vi "UpdateSpeeds.vi"(4 "SpeedMutiplier":dbl=2.0, 6 "Ramp (V/s)":dbl=2.0, 7 "robotPositionIn":T1, 8 "Enabled":bool=TRUE, 9 "Rotation (V)":dbl, 10 "Left/Right (V)":dbl, 11 "Forwards/Back (V)":dbl) -> (0 "M4 (V)":dbl, 1 "M3 (V)":dbl, 2 "M2 (V)":dbl, 3 "M1 (V)":dbl, 5 "robotPositionOut":T1)   [LabVIEW 2015]
panel:
  out "Distance Travelled (mm/0.01s)":dbl
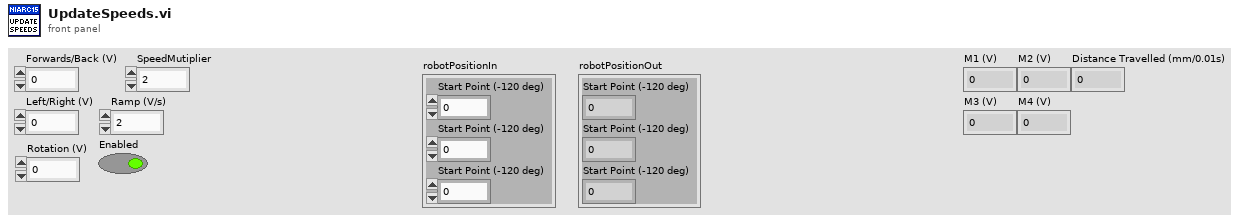
[diagram p1: front panel]
types:
  T1 = cluster{"Start Point (-120 deg)":dbl, "Start Point (-120 deg)":dbl, "Start Point (-120 deg)":dbl}
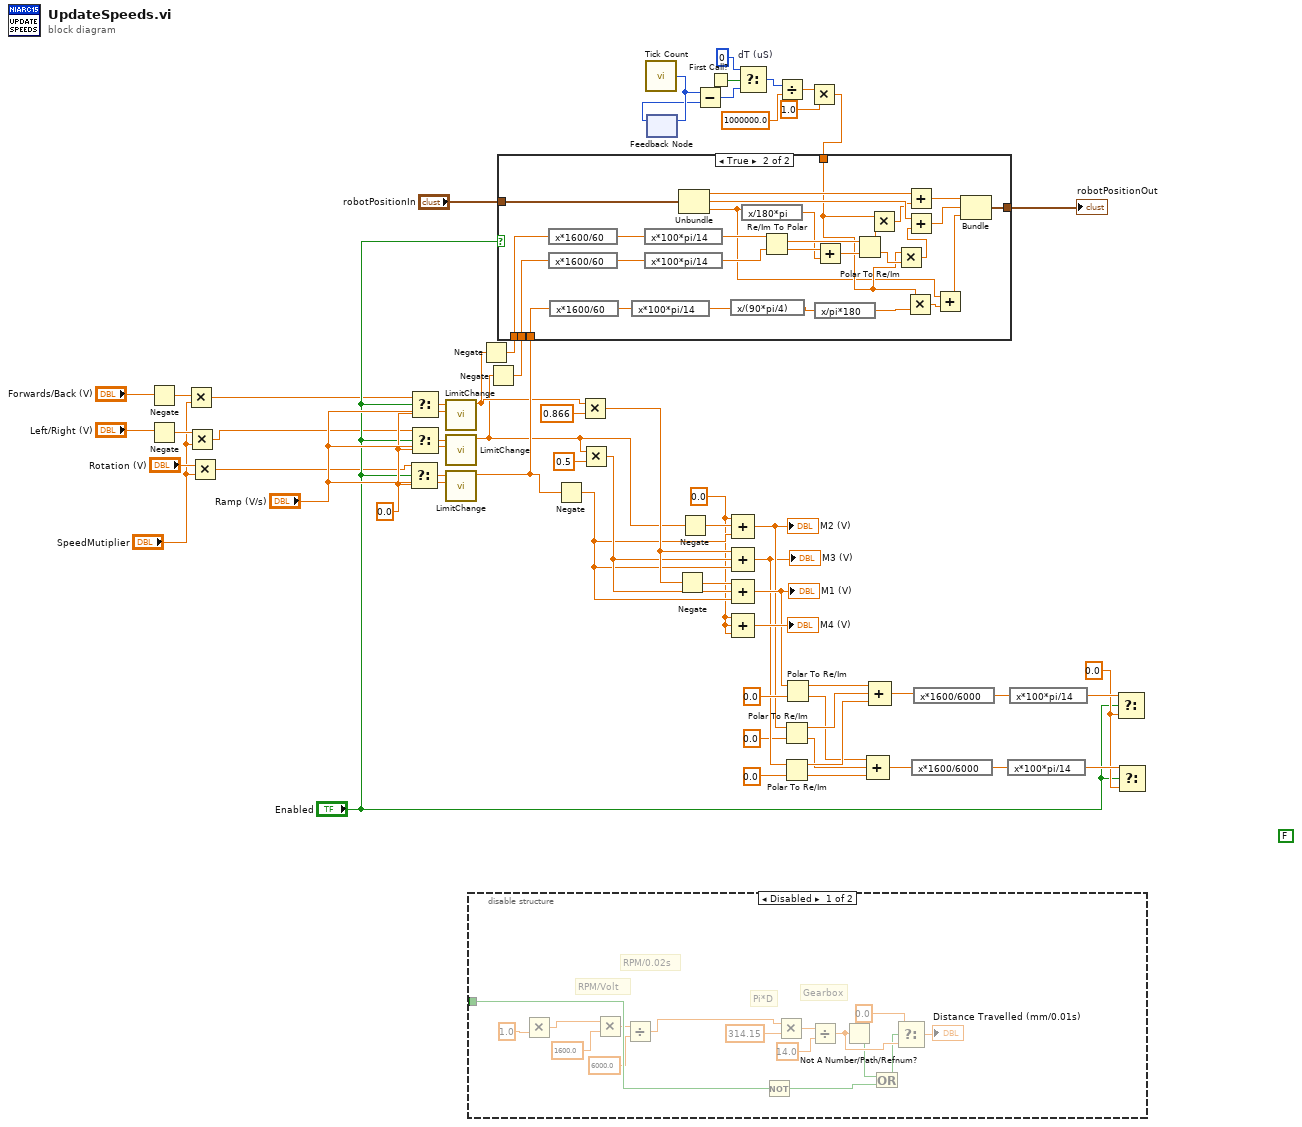
[diagram p0: block diagram]
diagram:
  (unwired) FALSE
  w26 = 0.0 ("f")
  w47 = 0.0 ("t")
  w55 = 0.0 ("f")
  n1 = Negate(x="Forwards/Back (V)") -> (-x=w10:dbl)
  n2 = Negate(x="Left/Right (V)") -> (-x=w9:dbl)
  n3 = Multiply(x=w10, y="SpeedMutiplier") -> (x*y=w6:dbl)
  n4 = Multiply(x=w9, y="SpeedMutiplier") -> (x*y=w5:dbl)
  n5 = Multiply(x="Rotation (V)", y="SpeedMutiplier") -> (x*y=w4:dbl)
  n6 = Select(t=w4, s="Enabled", f=w55) -> (s? t:f=w56:dbl)
  n7 = Select(t=w6, s="Enabled", f=w55) -> (s? t:f=w58:dbl)
  n8 = Select(t=w5, s="Enabled", f=w55) -> (s? t:f=w57:dbl)
  n9 = call "LimitChange.vi"("Ramp (1/s)"="Ramp (V/s)", "Set Point"=w58) -> ("Output"=w21:dbl)  [unwired: 9 in]
  n10 = call "LimitChange.vi"("Ramp (1/s)"="Ramp (V/s)", "Set Point"=w57) -> ("Output"=w20:dbl)  [unwired: 9 in]
  n11 = call "LimitChange.vi"("Ramp (1/s)"="Ramp (V/s)", "Set Point"=w56) -> ("Output"=w25:dbl)  [unwired: 9 in]
  n12 = disable-structure shown="Disabled" {
    disable-tunnel: _ -> [w67 _]
    frame Disabled {
      # "Gearbox"
      # "Pi*D"
      # "RPM/0.02s"
      # "RPM/Volt"
      n13 = Multiply(y=1.0) -> (x*y=w62:dbl)  [unwired: 1 in]
      n14 = Multiply(x=w62, y=1600.0) -> (x*y=w65:dbl)
      n15 = Divide(x=w65, y=6000.0) -> (x/y=w63:dbl)
      n16 = Not(x=w67) -> (.not. x?=w69:bool)
      n17 = Multiply(x=w63, y=314.15) -> (x*y=w75:dbl)
      n18 = Divide(x=w75, y=14.0) -> (x/y=w72:dbl)
      n19 = Not A Number/Path/Refnum?(number/path/refnum=w72) -> (NaN/Path/Refnum?=w70:bool)
      n20 = Or(x=w70, y=w69) -> (x .or. y?=w68:bool)
      n21 = Select(t=0.0, s=w68, f=w72) -> (s? t:f=→"Distance Travelled (mm/0.01s)":dbl)
    }
    frame Enabled {
    }
  }
  n22 = Negate(x=w21) -> (-x=w22:dbl)
  n23 = Negate(x=w20) -> (-x=w19:dbl)
  n24 = Negate(x=w25) -> (-x=w48:dbl)
  n25 = Multiply(x=w21, y=0.866) -> (x*y=w52:dbl)
  n26 = Multiply(x=w20, y=0.5) -> (x*y=w49:dbl)
  n27 = call "Tick Count"() -> ("Tick Count(uSec)"=w18:u32)
  n28 = feedback #1() -> (w17:u32)  [unwired: 1 in]
  n29 = feedback-in #1(w18) -> ()
  n30 = Negate(x=w52) -> (-x=w53:dbl)
  n31 = Negate(x=w20) -> (-x=w51:dbl)
  n32 = Subtract(x=w18, y=w17) -> (x-y=w15:u32)
  n33 = First Call?() -> (First Call?: T/F=w16:bool)
  n34 = Compound Arithmetic op=ADD(w47, w51, w48) -> (w42:dbl)
  "M2 (V)" <- w42
  n35 = Compound Arithmetic op=ADD(w52, w49, w48) -> (w41:dbl)
  "M3 (V)" <- w41
  n36 = Compound Arithmetic op=ADD(w53, w49, w48) -> (w44:dbl)
  "M1 (V)" <- w44
  n37 = Compound Arithmetic op=unknown(w47, w47, w47) -> (→"M4 (V)":dbl)
  n38 = Select "dT (uS)"(t=u32 0, s=w16, f=w15) -> (s? t:f=w13:u32)
  n39 = Divide(x=w13, y=1000000.0) -> (x/y=w3:dbl)
  n40 = Polar To Re/Im(2:0.0 ("theta"), 3:w42) -> (0:w33:dbl, 1:w36:dbl)
  n41 = Polar To Re/Im(2:0.0 ("theta"), 3:w41) -> (0:w32:dbl, 1:w35:dbl)
  n42 = Polar To Re/Im(2:0.0 ("theta"), 3:w44) -> (0:w34:dbl, 1:w37:dbl)
  n43 = Multiply(x=w3, y=1.0) -> (x*y=w1:dbl)
  n44 = case shown="True" "Enabled" {
    tunnel: w22 -> [_ w103]
    tunnel: w19 -> [_ w102]
    tunnel: w25 -> [_ w101]
    tunnel: "robotPositionIn" -> [w77 w98]
    tunnel: [w77 w86] -> w11
    tunnel: w1 -> [_ w81]
    frame False {
    }
    frame True {
      n45 = expression code="x*1600/60"(w103) -> (w106:dbl)
      n46 = expression code="x*1600/60"(w102) -> (w105:dbl)
      n47 = expression code="x*1600/60"(w101) -> (w104:dbl)
      n48 = expression code="x*100*pi/14"(w104) -> (w100:dbl)
      n49 = expression code="x*100*pi/14"(w106) -> (w97:dbl)
      n50 = expression code="x*100*pi/14"(w105) -> (w96:dbl)
      n51 = Unbundle(w98) -> ("Start Point (-120 deg)"=w91:dbl, "Start Point (-120 deg)"=w90:dbl, "Start Point (-120 deg)"=w78:dbl)
      n52 = expression code="x/(90*pi/4)"(w100) -> (w99:dbl)
      n53 = expression code="x/180*pi"(w78) -> (w92:dbl)
      n54 = Re/Im To Polar(2:w96, 3:w97) -> (0:w95:dbl, 1:w93:dbl)
      n55 = Add(x=w95, y=w92) -> (x+y=w94:dbl)
      n56 = expression code="x/pi*180"(w99) -> (w79:dbl)
      n57 = Polar To Re/Im(2:w94, 3:w93) -> (0:w85:dbl, 1:w84:dbl)
      n58 = Multiply(x=w81, y=w84) -> (x*y=w83:dbl)
      n59 = Multiply(x=w81, y=w85) -> (x*y=w82:dbl)
      n60 = Multiply(x=w81, y=w79) -> (x*y=w80:dbl)
      n61 = Add(x=w91, y=w83) -> (x+y=w89:dbl)
      n62 = Add(x=w90, y=w82) -> (x+y=w88:dbl)
      n63 = Add(x=w78, y=w80) -> (x+y=w87:dbl)
      n64 = Bundle(w89, w88, w87) -> (w86:cluster{dbl, dbl, dbl})  [unwired: 1 in]
    }
  }
  "robotPositionOut" <- w11
  n65 = Compound Arithmetic op=ADD(w34, w33, w32) -> (w29:dbl)
  n66 = Compound Arithmetic op=ADD(w37, w36, w35) -> (w31:dbl)
  n67 = expression code="x*1600/6000"(w29) -> (w30:dbl)
  n68 = expression code="x*1600/6000"(w31) -> (w38:dbl)
  n69 = expression code="x*100*pi/14"(w30) -> (w27:dbl)
  n70 = expression code="x*100*pi/14"(w38) -> (w28:dbl)
  n71 = Select(t=w28, s="Enabled", f=w26) -> ()  [unwired: 1 out]
  n72 = Select(t=w27, s="Enabled", f=w26) -> ()  [unwired: 1 out]
